vi "Get Record Length.vi"(0 "Time (s)":dbl, 5 "Sample Rate":dbl) -> (4 "Record Length":dbl)   [LabVIEW 2020, in "LDO Load Transient_AWG.lvlib"]
uses:
  LDO Load Transient_AWG.lvlib
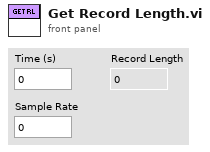
[diagram p1: front panel]
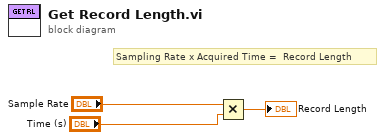
[diagram p0: block diagram]
diagram:
  # "Sampling Rate x Acquired Time =  Record Length"
  n1 = Multiply(x="Sample Rate", y="Time (s)") -> (x*y=→"Record Length":dbl)
